vi "Init Pattern Parser.vi"(9 "Options":T1, 10 "Encoding Callback":refnum<vi>, 11 "Input":string) -> (0 "error out":errorcluster, 3 "Pattern Parser":T2)   [LabVIEW 2020, in "Stream.lvlib" / "URLPattern.lvclass"]
uses:
  URLPattern.lvclass
  Token Type.ctl
  Token.ctl
  Pattern Part Type.ctl
  Pattern Part Modifier.ctl
  Pattern Part.ctl
  Pattern Parser.ctl
  Tokenize Policy.ctl
  Pattern String Options.ctl
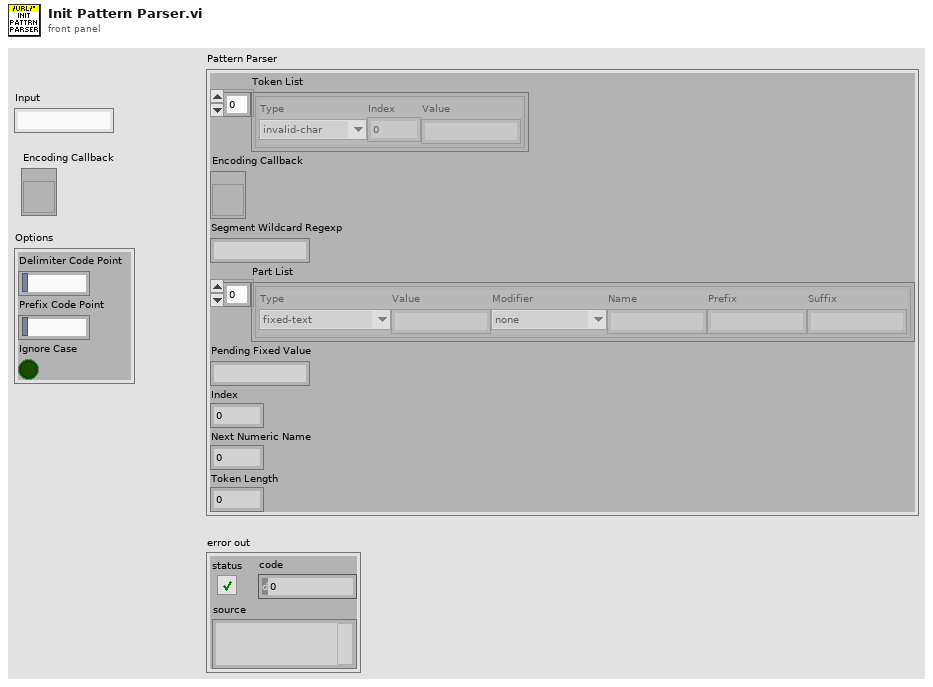
[diagram p1: front panel]
types:
  T1 = typedef "Stream.lvlib/URLPattern.lvclass/Pattern String Options.ctl" = cluster{"Delimiter Code Point":string, "Prefix Code Point":string, "Ignore Case":bool}
  T2 = typedef "Stream.lvlib/URLPattern.lvclass/Pattern Parser.ctl" = cluster{"Token List":T3[], "Encoding Callback":refnum<vi>, "Segment Wildcard Regexp":string, "Part List":T5[], "Pending Fixed Value":string, "Index":i32, "Next Numeric Name":i32, "Token Length":i32}
  T3 = typedef "Stream.lvlib/URLPattern.lvclass/Token.ctl" = cluster{"Type":T4, "Index":i32, "Value":string}
  T4 = typedef "Stream.lvlib/URLPattern.lvclass/Token Type.ctl" = enum16{"invalid-char", "open", "close", "regexp", "name", "char", "escaped-char", "other-modifier", "asterisk", "end"}
  T5 = typedef "Stream.lvlib/URLPattern.lvclass/Pattern Part.ctl" = cluster{"Type":T6, "Value":string, "Modifier":T7, "Name":string, "Prefix":string, "Suffix":string}
  T6 = typedef "Stream.lvlib/URLPattern.lvclass/Pattern Part Type.ctl" = enum16{"fixed-text", "regexp", "segment-wildcard", "full-wildcard"}
  T7 = typedef "Stream.lvlib/URLPattern.lvclass/Pattern Part Modifier.ctl" = enum16{"none", "optional", "zero-or-more", "one-or-more"}
  T8 = typedef "Stream.lvlib/URLPattern.lvclass/Tokenize Policy.ctl" = enum16{"strict", "lenient"}
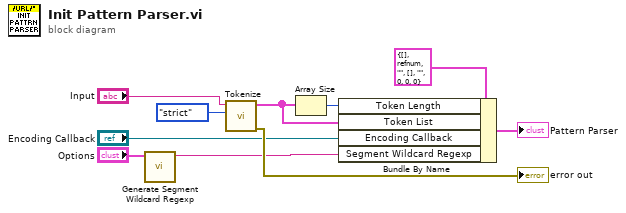
[diagram p0: block diagram]
diagram:
  n1 = call "Generate Segment Wildcard Regexp.vi"("Options"="Options") -> ("Segment Wildcard Regexp"=w6:string)  [unwired: 10 in]
  n2 = call "Tokenize.vi"("Policy"=Tokenize_Policy."strict", "Input"="Input") -> ("error out"=→"error out":errorcluster, "Token List"=w3:T3[])  [unwired: 8 in]
  n3 = Array Size(array=w3) -> (size(s)=w2:i32)
  n4 = Bundle By Name(cluster=T2 {"Token List"=[], "Encoding Callback"=refnum, "Segment Wildcard Regexp"="", "Part List"=[], "Pending Fixed Value"="", "Index"=0, "Next Numeric Name"=0, "Token Length"=0} ("Pattern Parser"), "Token Length"=w2, "Token List"=w3, "Encoding Callback"="Encoding Callback", "Segment Wildcard Regexp"=w6) -> (→"Pattern Parser":T2)
